vi "setVerticalCoupling.vi"(7 "Channel Name (0: Channel 1)":i32(ring) items=["Channel 1", "Channel 2", "Channel 3", "Channel 4"], 8 "error in (no error)":errorcluster, 9 "Coupling (1: DC)":i32(ring)=1 items=["AC", "DC"], 10 "Impedance (0: 1 MOhm)":i32(ring) items=["1 MOhm", "50 Ohm"], 11 "VISA resource name":refnum<visa-resource-name>) -> (0 "error out":errorcluster, 3 "VISA resource name out":refnum<visa-resource-name>)   [LabVIEW 2023, in "Keysight-DSQx3014T.lvlib"]
doc: "<b>Author:</b> Wolfgang\n<b>Description:</b> Configures Vertical Coupling"
uses:
  Keysight-DSQx3014T.lvlib
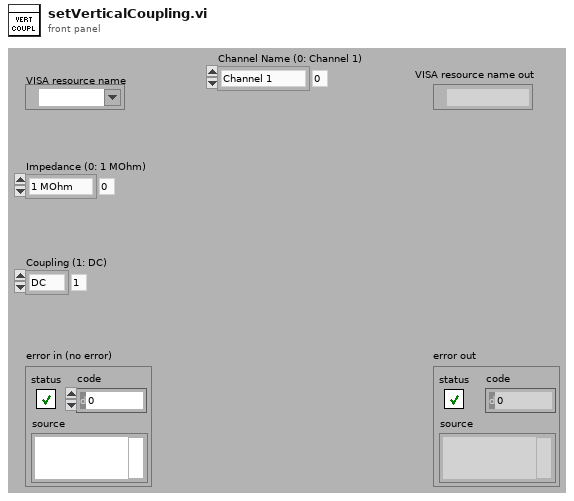
[diagram p1: front panel]
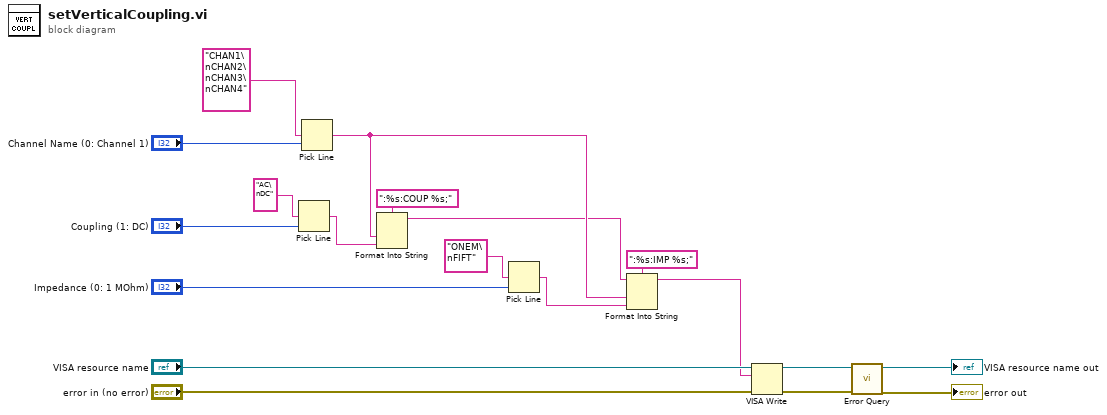
[diagram p0: block diagram]
diagram:
  n1 = Pick Line(multi-line string="AC\nDC", line index="Coupling (1: DC)") -> (output string=w16:string)  [unwired: 1 out]
  n2 = Pick Line(multi-line string="CHAN1\nCHAN2\nCHAN3\nCHAN4", line index="Channel Name (0: Channel 1)") -> (output string=w3:string)  [unwired: 1 out]
  n3 = Format Into String(format string=":%s:COUP %s;", w3, w16) -> (resulting string=w1:string)  [unwired: 2 in, 1 out]
  n4 = Pick Line(multi-line string="ONEM\nFIFT", line index="Impedance (0: 1 MOhm)") -> (output string=w12:string)  [unwired: 1 out]
  n5 = Format Into String(format string=":%s:IMP %s;", initial string=w1, w3, w12) -> (resulting string=w2:string)  [unwired: 1 in, 1 out]
  n6 = VISA Write(VISA resource name="VISA resource name", write buffer=w2, error in (no error)="error in (no error)") -> (VISA resource name out=w9:refnum<visa-resource-name>, error out=w8:errorcluster)  [unwired: 1 out]
  n7 = call "Error Query.vi"("error in (no error)"=w8, "VISA resource name"=w9) -> ("error out"=→"error out":errorcluster, "VISA resource name out"=→"VISA resource name out":refnum<visa-resource-name>)  [unwired: 8 out]
